vi "Close Items.vi"(11 "Tree in":refnum<class "Tree.lvclass">) -> (3 "Tree out":refnum<class "Tree.lvclass">)   [LabVIEW 2022 SP3, in "Tree.lvclass"]
uses:
  Tree.lvclass
  Tree.lvclass/Tree.ctl
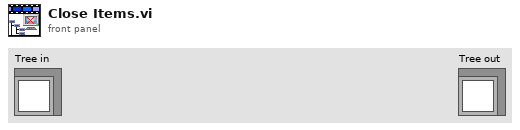
[diagram p1: front panel]
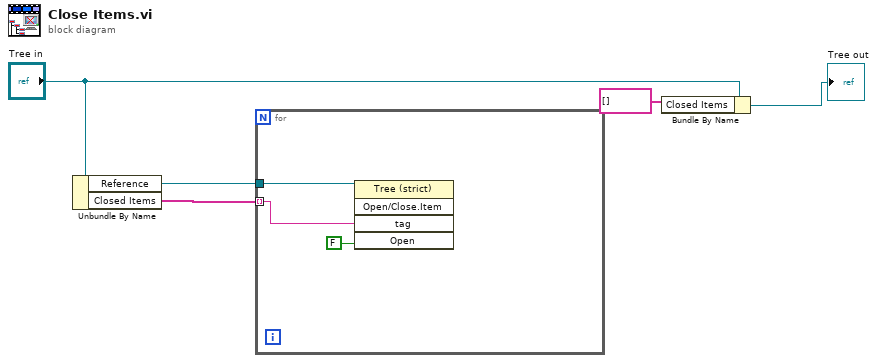
[diagram p0: block diagram]
diagram:
  n1 = Unbundle By Name("Tree in") -> ("Reference"=w4:refnum<vi>, "Closed Items"=w5:string[])
  n2 = for {
    tunnel: w5 -> [w7] mode=indexing
    tunnel: w4 -> [w8]
    n3 = invoke class="Tree (strict)" method="Open/Close.Item"(reference=w8, "tag"=w7, "Open"=FALSE ("Open?")) -> ()  [unwired: 2 in, 5 out]
  }
  n4 = Bundle By Name(cluster="Tree in", "Closed Items"=string[] []) -> (→"Tree out":refnum<class "Tree.lvclass">)
